vi "After Launch Init.vi"(8 "error in (no error)":errorcluster, 11 "HIJ Vision Camera App in":refnum<class "HIJ Vision Camera App.lvclass">) -> (0 "error out":errorcluster, 3 "HIJ Vision Camera App out":refnum<class "HIJ Vision Camera App.lvclass">)   [LabVIEW 2014, in "HIJ Vision Camera App.lvlib" / "HIJ Vision Camera App.lvclass"]
uses:
  HIJ Vision Camera App.lvclass
  Display Actors/HIJ Vision Display/HIJ Vision Display Messages/New Image Msg/New Image Msg.lvclass
  HIJ Vision Application/HIJ Vision Application/HIJ Vision Application.lvclass/HIJ Vision Application.ctl
  HIJ Vision Camera App.lvclass/HIJ Vision Camera App.ctl
  Camera Actors/Camera Actor/Camera Actor Messages/Write Receiver Params Msg/Write Receiver Params Msg.lvclass/Write Receiver Params Msg.ctl
  <vilib>/ActorFramework/Message Enqueuer/Message Enqueuer.lvclass/Message Enqueuer.ctl
  HIJ Vision Application/HIJ Vision Application/Read Display Enq.vi
  <vilib>/ActorFramework/Message Enqueuer/Enqueue.vi
  <vilib>/ActorFramework/Message Priority Queue/Priority Enqueue.vi
  HIJ Vision Application/HIJ Vision Application/HIJ Vision Application.lvclass
  <vilib>/ActorFramework/Message Enqueuer/Message Enqueuer.lvclass
  Camera Actors/Camera Actor/Camera Actor Messages/Write Receiver Params Msg/Write Receiver Params Msg.lvclass
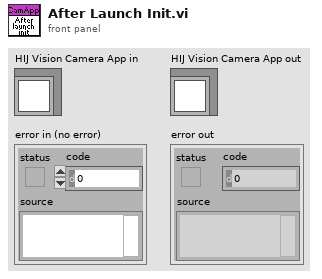
[diagram p1: front panel]
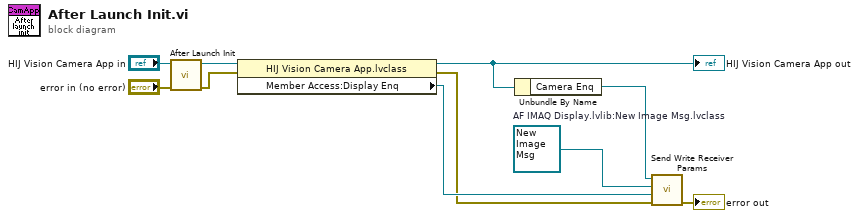
[diagram p0: block diagram]
diagram:
  w5 = refnum<class "New Image Msg.lvclass"> refnum  # AF IMAQ Display.lvlib:New Image Msg.lvclass
  n1 = call-parent "After Launch Init.vi"("error in (no error)"="error in (no error)", "HIJ Vision Application in"="HIJ Vision Camera App in") -> ("error out"=w3:errorcluster, "HIJ Vision Application out"=w10:refnum<class "HIJ Vision Camera App.lvclass">)  [unwired: 8 in]
  n2 = property class="HIJ Vision Camera App.lvclass"(reference=w10, error in=w3) -> (reference out=w7:refnum<class "HIJ Vision Camera App.lvclass">, error out=w2:errorcluster, "Member Access:Display Enq"=w4:refnum<class "Message Enqueuer.lvclass">)
  "HIJ Vision Camera App out" <- w7
  n3 = Unbundle By Name(w7) -> ("Camera Enq"=w6:refnum<class "Message Enqueuer.lvclass">)
  n4 = call "Send Write Receiver Params.vi"("error in (no error)"=w2, "Image Receiver"=w4, "New Image Msg"=w5, "Message Enqueuer"=w6) -> ("error out"=→"error out":errorcluster)  [unwired: 6 in, 1 out]
